vi "Get New Level.vi"(8 "error in (no error)":errorcluster, 11 "Level Controller in":refnum<class "Level Controller.lvclass">) -> (0 "error out":errorcluster, 2 "Level":dbl, 3 "Level Controller out":refnum<class "Level Controller.lvclass">)   [LabVIEW 2018, in "Level Controller.lvlib" / "Level Controller.lvclass"]
doc: "This VI specifies what variable the level controller is monitoring. When called, this VI should return the current value of that variable. Child classes must override this method."
uses:
  Level Controller.lvclass
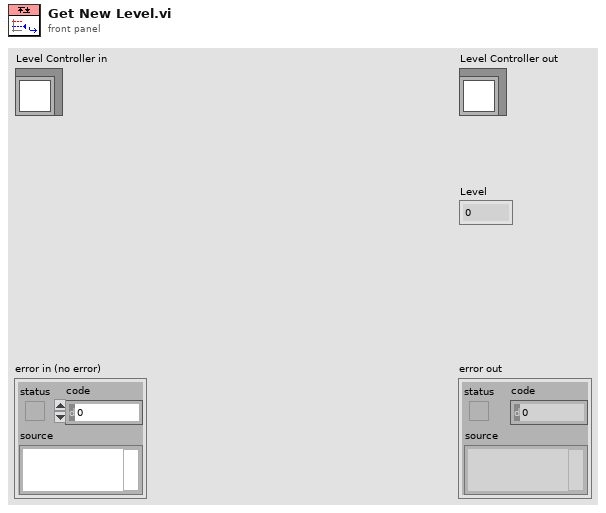
[diagram p1: front panel]
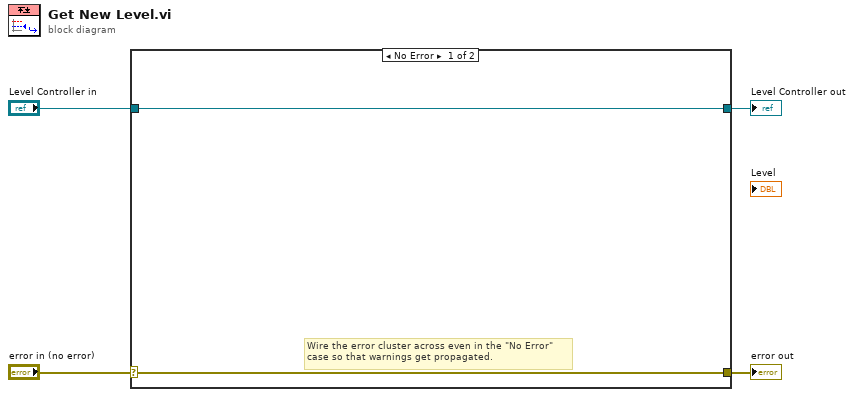
[diagram p0: block diagram]
diagram:
  n1 = case shown="No Error" "error in (no error)" {
    selector: "error in (no error)" -> [w5 w8]
    tunnel: [w5 w8] -> w3
    tunnel: [w6 w7] -> w1
    tunnel: "Level Controller in" -> [w6 w7]
    frame No Error {
      # "Wire the error cluster across even in the \"No Error\"\ncase so that warnings get propagated."
    }
    frame Error {
    }
  }
  "error out" <- w3
  "Level Controller out" <- w1
